vi "XNET Read (Frame Ethernet).vi"(0 "session in":refnum<k21>, 7 "number to read (-1)":i32=-1, 9 "timeout (0)":dbl format="%.2g", 11 "error in (no error)":errorcluster) -> (4 "session out":refnum<k21>, 6 "data":T1[](array[typedef]) {"fcs" format="%08x"; "network timestamp" format="%<%.7X\n%x>T"; "frame data" format="%x"; "local timestamp" format="%<%.7X\n%x>T"; "type" items=["Ethernet Data"=0, "Delay"=225, "Future Time Wait"=226]}, 14 "unused payloads":cluster{"payload":u8[]}[](array[cluster]), 15 "error out":errorcluster)   [LabVIEW 2018]
doc: "Reads data from a session as an array of Ethernet frames. The session must use an Ethernet interface and a mode of Frame Input Stream."
uses:
  XNET Frame Ethernet.ctl
  XNET Frame Type Ethernet.ctl
  nixlvapi.dll
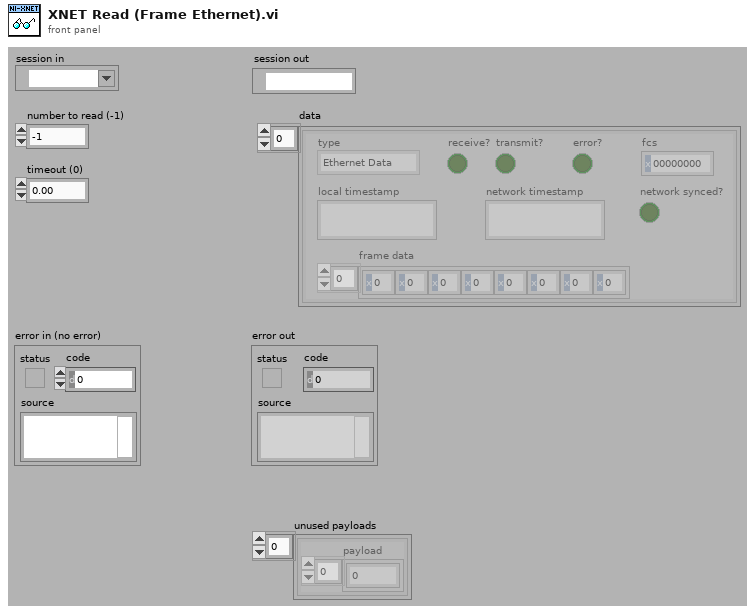
[diagram p1: front panel]
types:
  T1 = typedef "XNET Frame Ethernet.ctl" = cluster{"local timestamp":timestamp, "network timestamp":timestamp, "frame data":u8[], "fcs":u32, "type":T2, "network synced?":bool, "receive?":bool, "transmit?":bool, "error?":bool}
  T2 = typedef "XNET Frame Type Ethernet.ctl" = u16
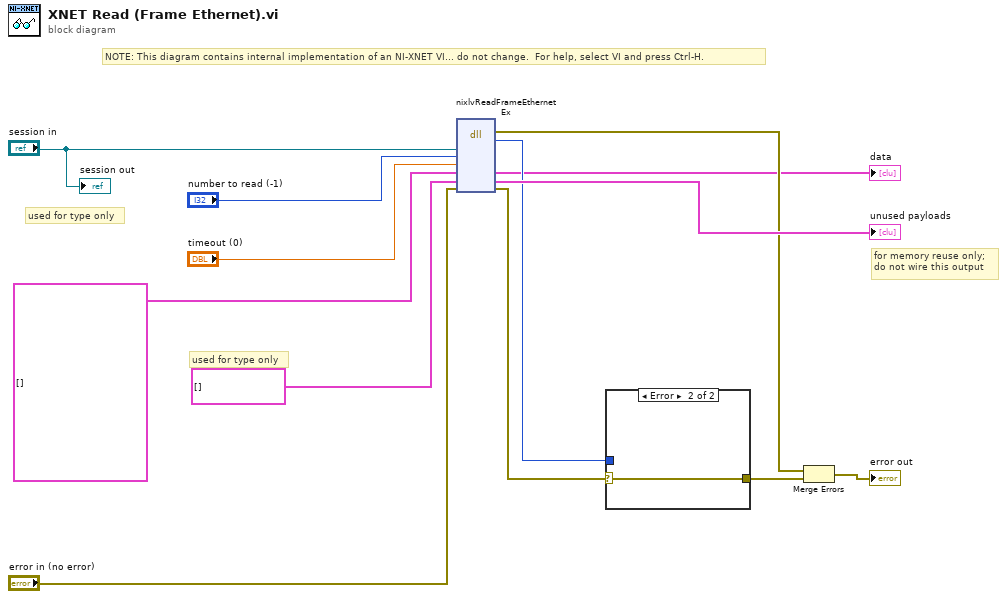
[diagram p0: block diagram]
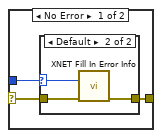
[diagram p2: hidden frame]
diagram:
  # "for memory reuse only;\ndo not wire this output"
  # "used for type only"
  # "used for type only"
  # "NOTE: This diagram contains internal implementation of an NI-XNET VI... do not change.  For help, select VI and press Ctrl-H."
  n1 = dll-call lib="nixlvapi.*" fn="nixlvReadFrameEthernetEx" label="Call Library"("sessionRef"="session in", "numberToRead"="number to read (-1)", "timeout"="timeout (0)", "lvData"=T1[] [] ("data"), "unusedPayloads"=cluster{"payload":u8[]}[] [] ("payload array"), "errorInOut"="error in (no error)") -> (error out=w3:errorcluster, "return type"=w6:i32, "lvData"=→"data":T1[], "unusedPayloads"=→"unused payloads":cluster{"payload":u8[]}[], "errorInOut"=w5:errorcluster)  [unwired: 5 in, 2 out]
  n2 = case shown="Error" w5 {
    selector: w5 -> [w14 w21]
    tunnel: [w16 w21] -> w13
    tunnel: w6 -> [w15 _]
    frame No Error {
      n3 = case shown="Default" w15 {
        selector: w15 -> [_ w18]
        tunnel: w14 -> [w17 w19]
        tunnel: [w17 w20] -> w16
        frame 0 {
        }
        frame Default {
          n4 = call "XNET Fill In Error Info.vi"("status code"=w18, "error in"=w19) -> ("error out"=w20:errorcluster)  [unwired: 13 out]
        }
      }
    }
    frame Error {
    }
  }
  n5 = Merge Errors(w3, w13) -> (→"error out":errorcluster)
  "session out" <- "session in"
